vi "initScale.vi"(8 "error in (no error)":errorcluster, 11 "Scale Emulator in":refnum<class "Scale Emulator.lvclass">) -> (0 "error out":errorcluster, 3 "Scale Emulator out":refnum<class "Scale Emulator.lvclass">)   [LabVIEW 2015, in "Scale Emulator.lvclass"]
uses:
  Scale Emulator.lvclass
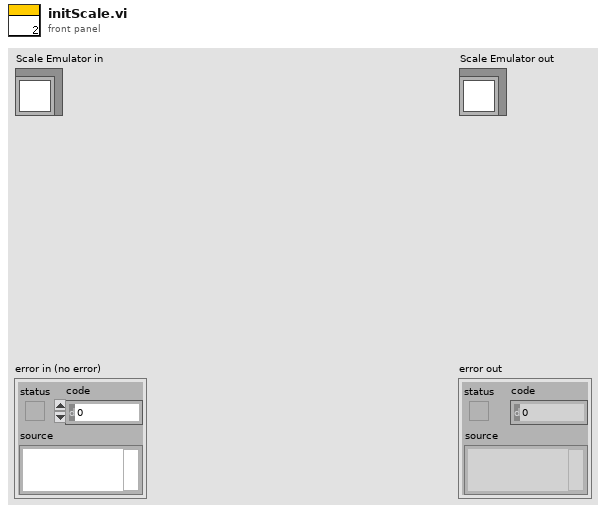
[diagram p1: front panel]
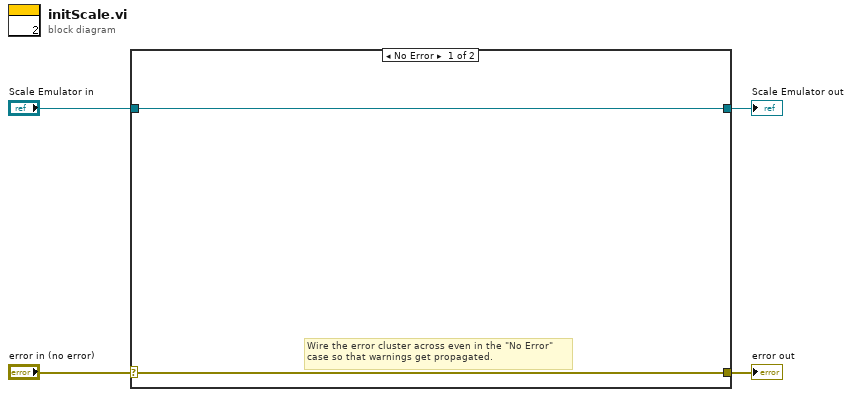
[diagram p0: block diagram]
diagram:
  n1 = case shown="No Error" "error in (no error)" {
    selector: "error in (no error)" -> [w5 w8]
    tunnel: [w5 w8] -> w3
    tunnel: [w6 w7] -> w1
    tunnel: "Scale Emulator in" -> [w6 w7]
    frame No Error {
      # "Wire the error cluster across even in the \"No Error\"\ncase so that warnings get propagated."
    }
    frame Error {
    }
  }
  "error out" <- w3
  "Scale Emulator out" <- w1
